vi "PS_Main.vi"() -> ()   [LabVIEW 2011]
uses:
  PS_Global.vi
  <vilib>/express/express shared/transition.llb/Dynamic To Waveform Array.vi
  <vilib>/express/express shared/transition.llb/Waveform Array To Dynamic.vi
  <vilib>/express/express arith-compare/Formula/Block/exnFormulaBlock how many pts in the wave.vi
  <vilib>/express/express shared/ex_Modify Signal Name.vi
  <vilib>/express/express arith-compare/Formula/XNode/ExpressFormulaBlockNode.xnode
panel:
  out "Std":dbl format="%#.2g%"
  out "New Value":dbl
  out "Counter":i32=1000
  out "Numbers to Avg":dbl[](array[numeric])
  in  "# in avg":i32=1000
  in  "Init Running Avg":bool
  out "Running Average":dbl format="%#.1f%"
  in  "New Discharge ON":bool
  in  "Pressure Calib":dbl=0.553
  out "LCR V Min":dbl
  in  "Discharge Voltage":dbl=10.3
  in  "Cell Pressure":dbl
  out "LCR Min V":dbl
  out "LCR Max V":dbl
  in  "stop":bool
  out "Heartbeat":string
  in  "Set All Offsets":bool
  in  "Run Polarimeter?":bool=TRUE
  out "Laser Peak Progress":i32(slide) scale=0.0..100.0
  out "Laser Global":bool
  in  "C8 Line?":bool caption="Laser State"
  out "LCR Calibration Plot":cluster{"Y":dbl[], "Y":dbl[]}[](graph)
  in  "Lower Voltge Limit":dbl=1.2
  in  "Upper Voltage Limit":dbl=4.0
  in  "Polarimeter Angle":dbl=20.0
  in  "CP In?":bool
  in  "Comment Box":string
  in  "Insert Comment":bool
  in  "Plasma On Length":dbl=0.2
  in  "Calibrate LCR":bool
  out "Plasma On":dbl
  out "Plasma State":bool caption="Plasma Ball Status"
  out "Plasma On":timestamp
  out "Shutter Closed":dbl format="%.0f sec"
  out "Shutter Time":timestamp
  in  "Shutter Set":bool=TRUE
  out "Shutter State":bool=TRUE caption="Shutter Status"
  out "log":refnum<file>
  out "VI Running":bool
  out "Off Time":timestamp
  out "On Time":timestamp
  out "Discharge State":bool caption="Discharge Status"
  out "Decay Running":bool caption="Status"
  out "Start Time":timestamp
  out "Duration":dbl
  in  "Discharge Interval":dbl=30.0
  in  "Discharge Length":dbl=5.0
  in  "Run Decay":bool
  in  "Discharge Set":bool
  out "Nuclear Polarization":dbl format="%#.1f%"
  out "Messages":string
  out "Corrected Low":dbl
  out "Corrected High":dbl
  out "Signal Offset: Laser Off":dbl
  in  "Laser State Set":bool caption="Laser State"
  out "Signal Offset: Laser On":dbl
  in  "Get Signal Offset":bool
  in  "High Signal Extend":i32
  out "Std Dev Low":dbl format="%.5f"
  out "Std Dev High":dbl format="%.5f"
  out "Optical Polarization (%)":dynamicdata(graph)
  out "Optical Polarization":dbl format="%#.1f%"
  out "Signals":dynamicdata(graph) caption="Section"
  out "Mean Low":dbl format="%.4f"
  out "Mean High":dbl format="%.4f"
  in  "High Signal Start":i32=600 caption="Begin Sample"
  in  "Low Signal Start":i32=600 caption="Begin Sample"
  out "Status":string
  out "Laser Peaks":cluster{dbl[], dbl[]}[](graph)
  out "Laser Peak Voltage Set":dbl format="%#_g V"
  in  "Run Laser Peak Find":bool
  in  "Number of Samples":i32=1000
  in  "Sample Rate (Hz)":dbl=4000.0
  # "Set Laser State"
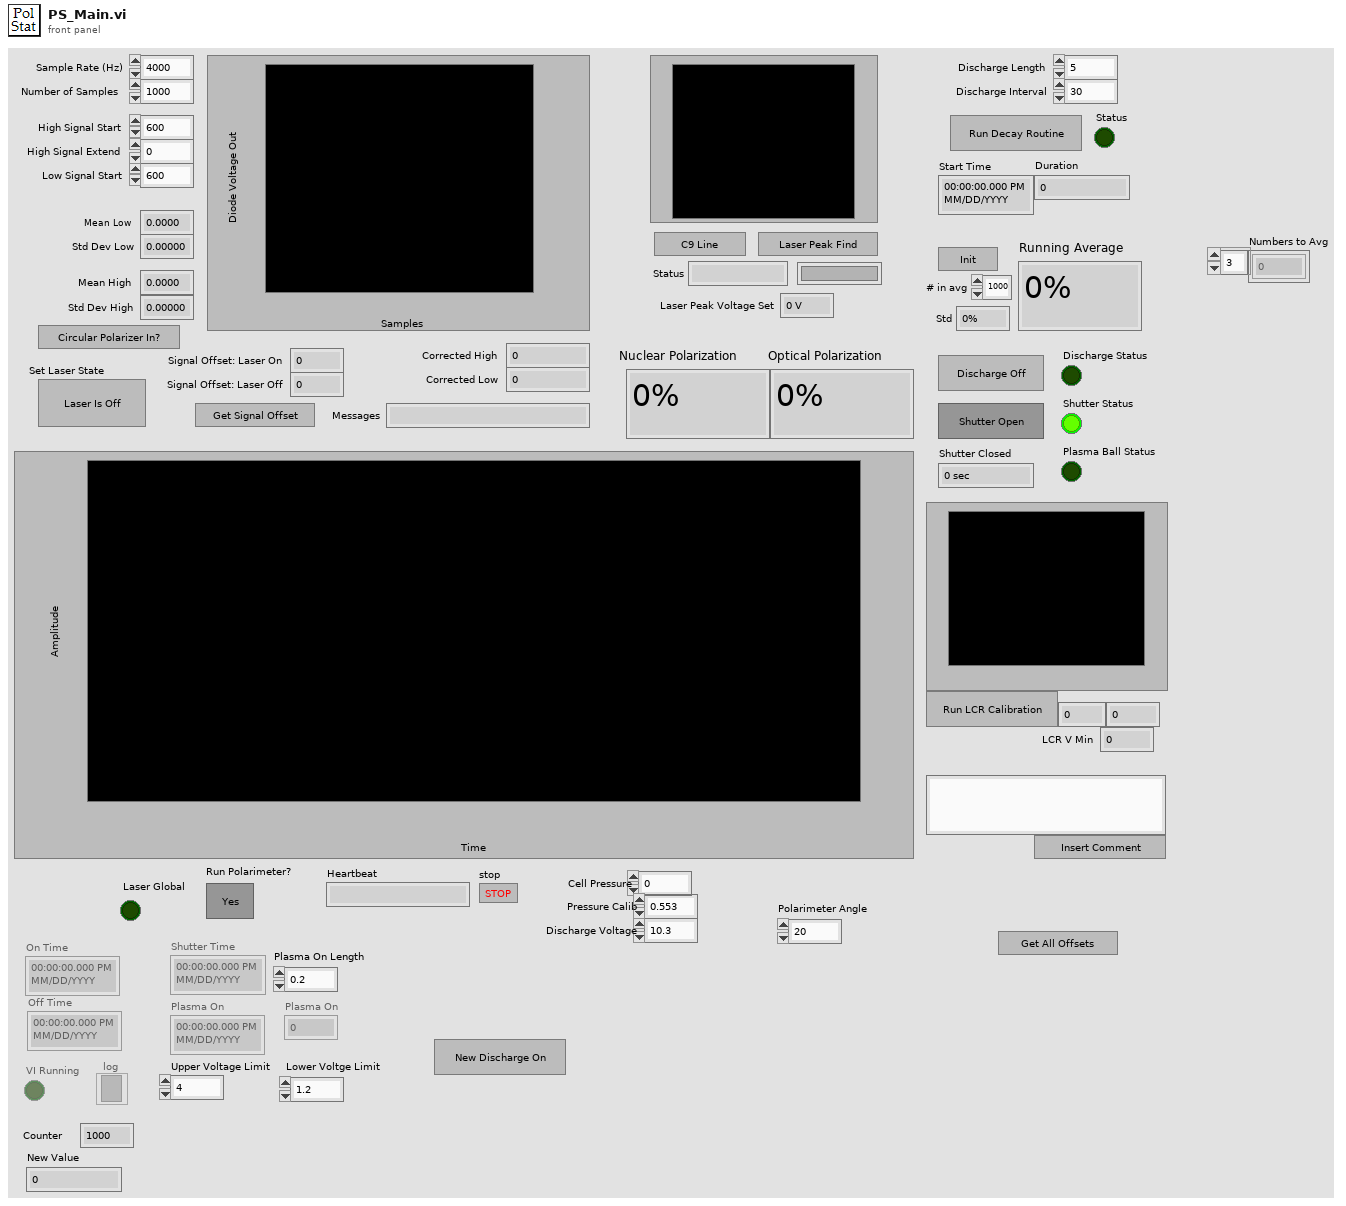
[diagram p1: front panel]
types:
  T1 = enum16{"open", "replace", "create", "open or create", "replace or create", "replace or create with confirmation"}
  T2 = enum8{"Enabled", "Disabled", "Disabled and Grayed Out"}
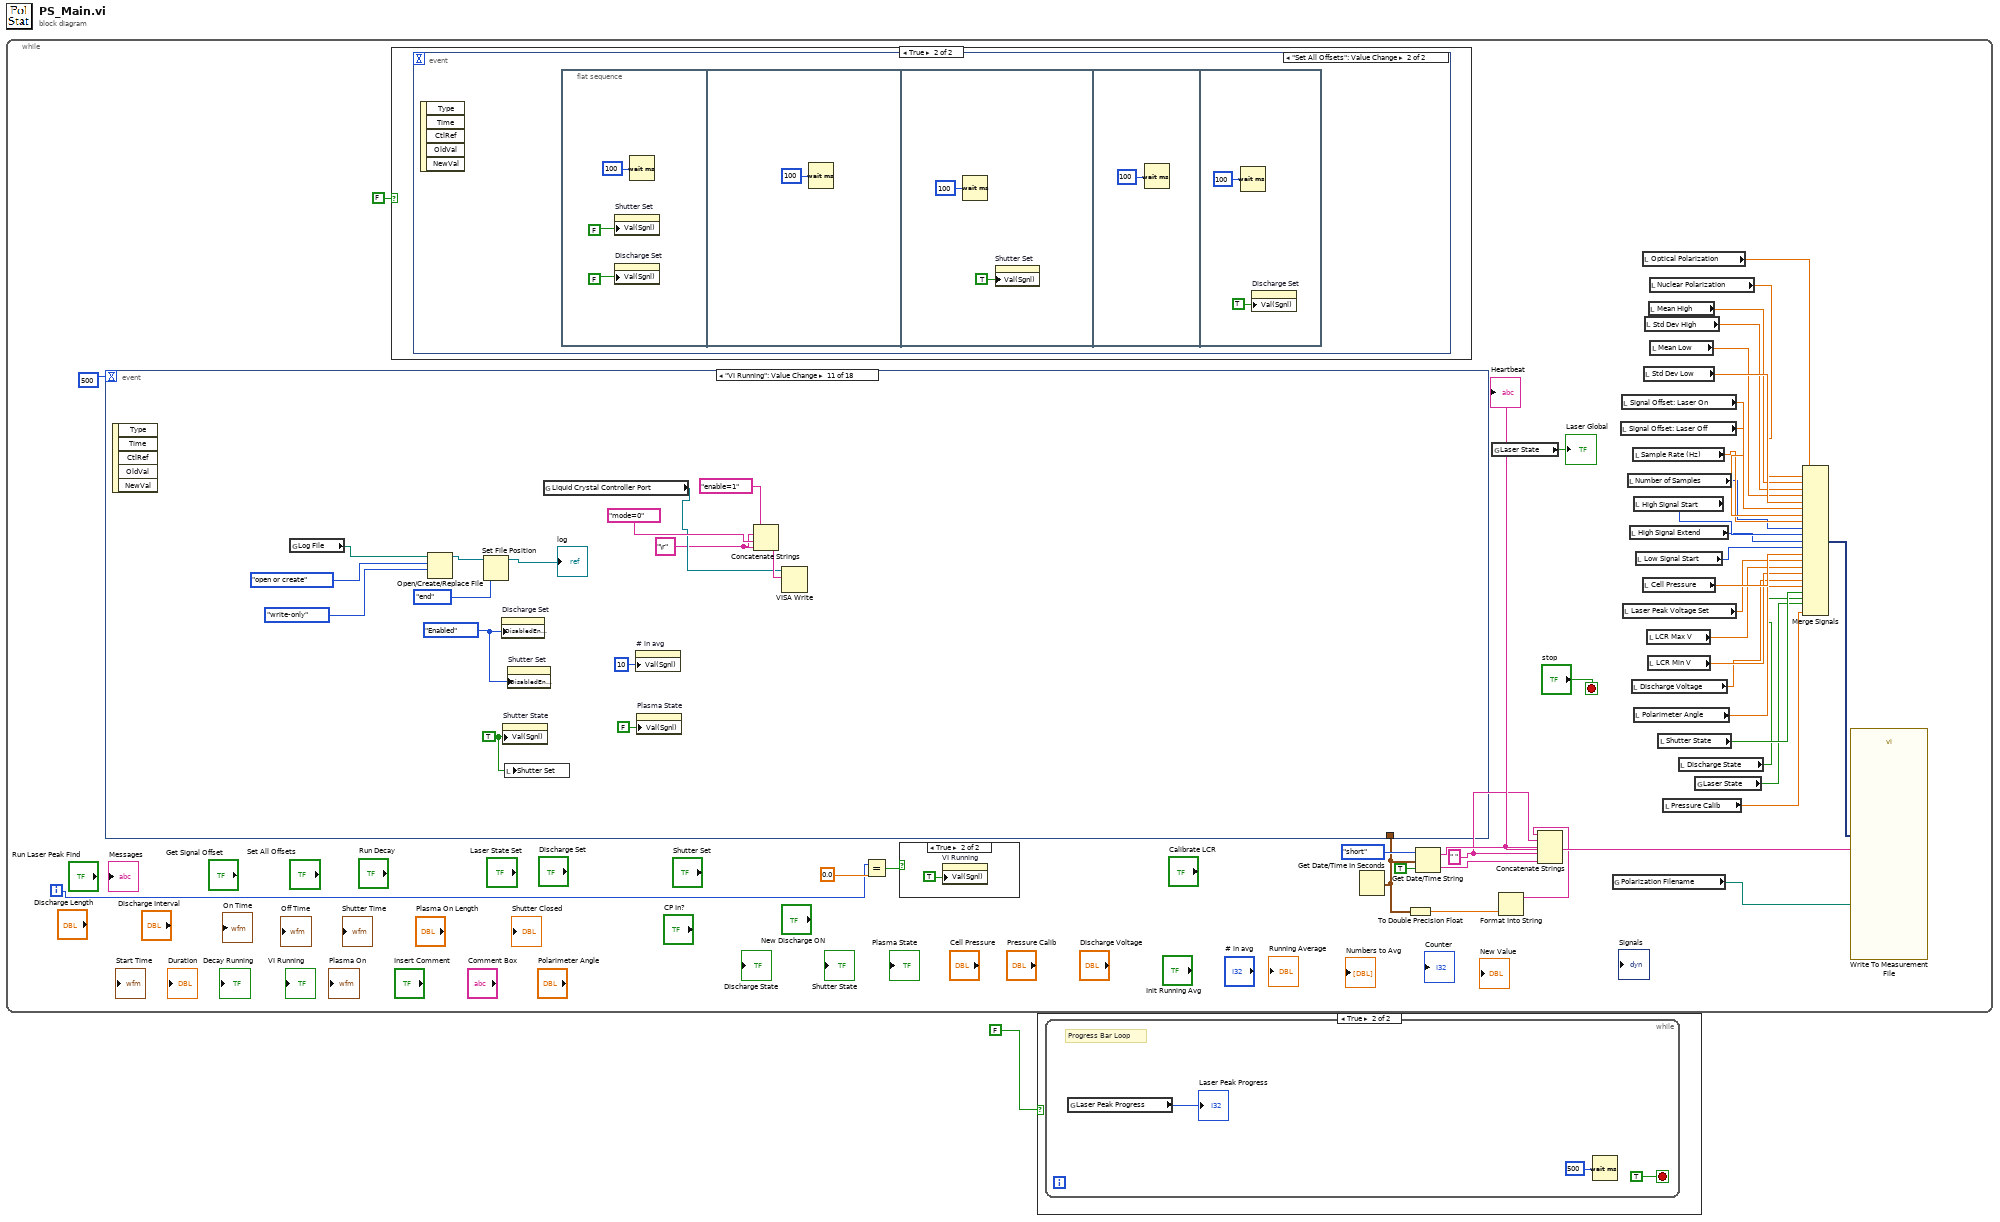
[diagram p0: block diagram]
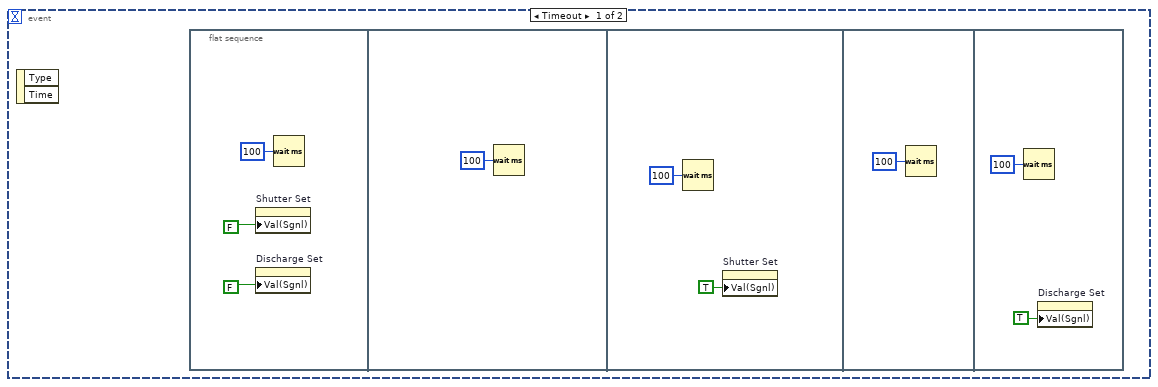
[diagram p4: hidden frame]
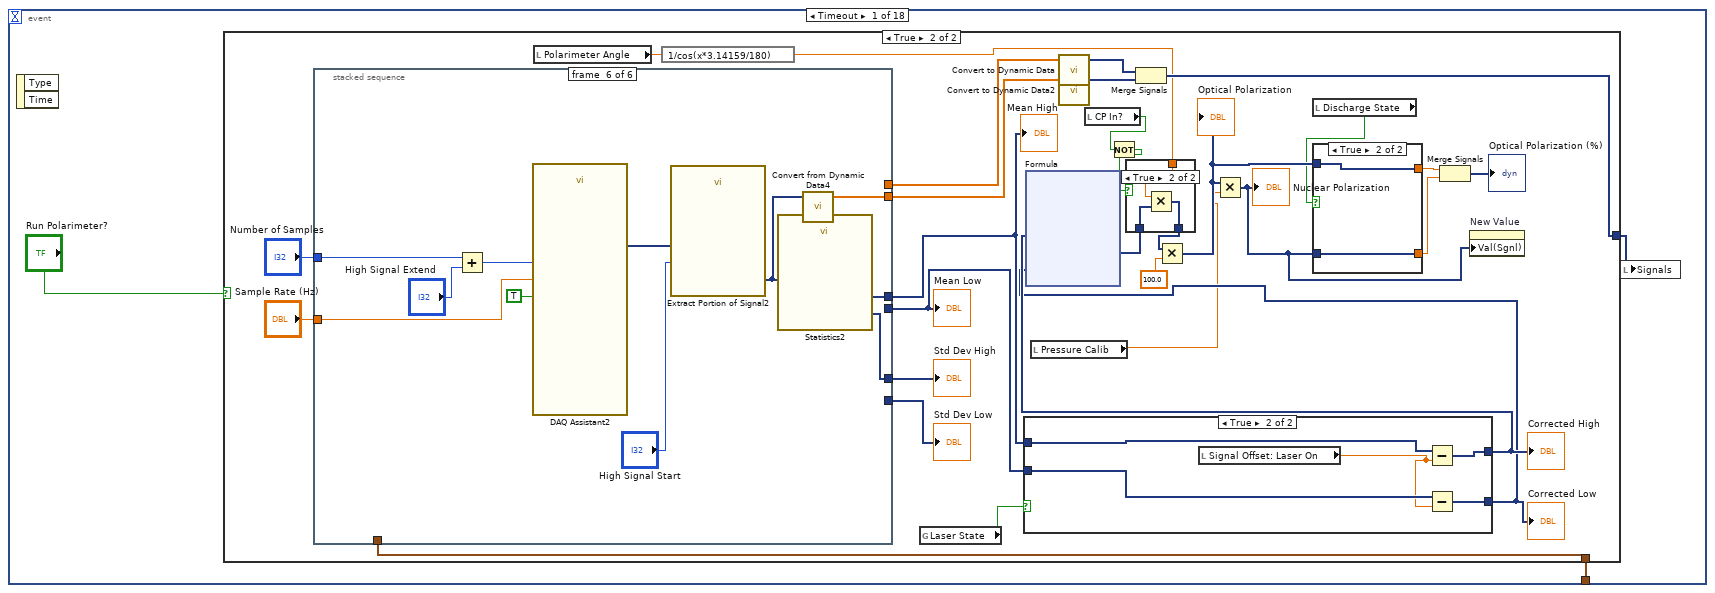
[diagram p6: hidden frame]
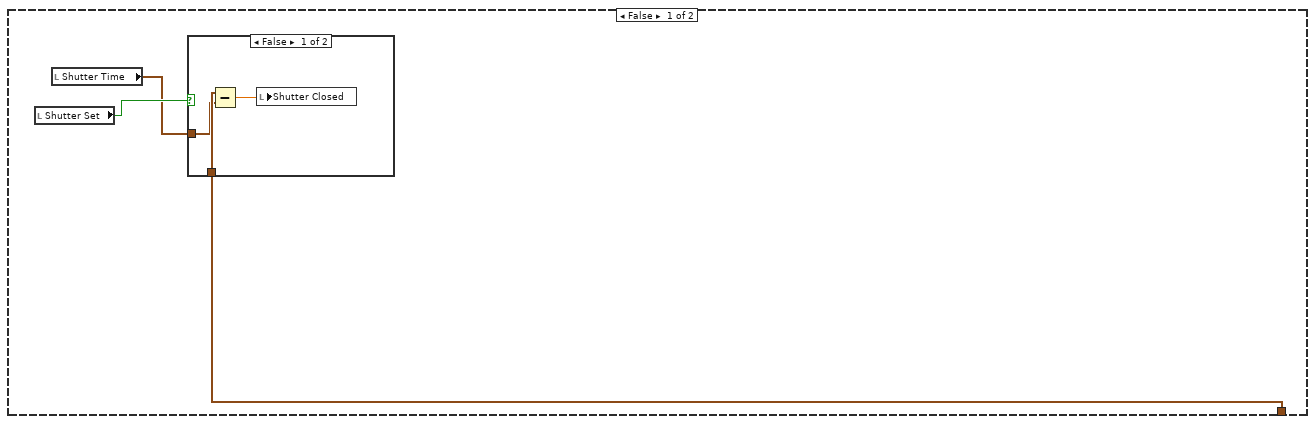
[diagram p7: hidden frame]
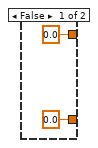
[diagram p9: hidden frame]
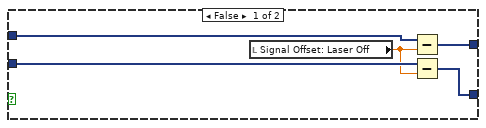
[diagram p11: hidden frame]
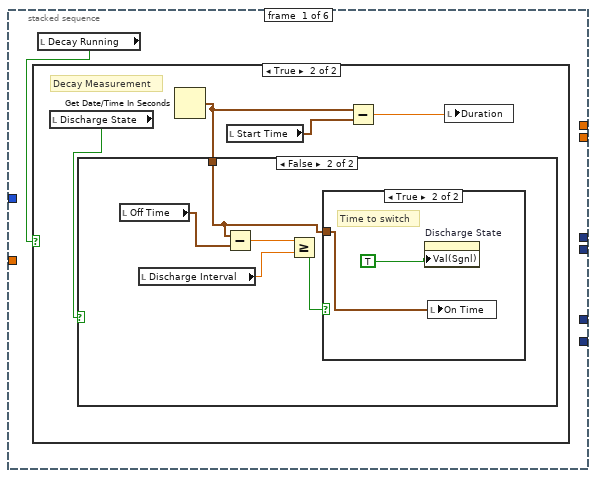
[diagram p12: hidden frame]
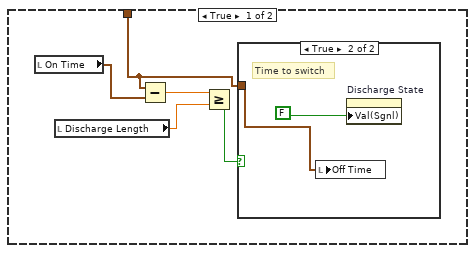
[diagram p14: hidden frame]
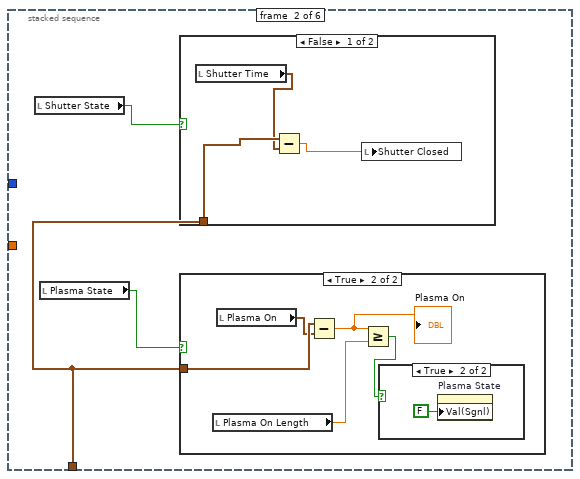
[diagram p17: hidden frame]
diagram:
  n1 = while {
    i -> [w34]
    stop <- "stop" stop-if-true
    w6 = " " ("string")
    n2 = case shown="True" FALSE {
      frame False {
      }
      frame True {
        n3 = event shown="[1] \"Set All Offsets\": Value Change" {
          selector: _ -> [_ _]
          dyn-events: _ -> [_ _]
          timeout: _ -> [_ _]
          event Timeout {
            n4 = event-data() -> ()  [unwired: 1 in, 2 out]
            n5 = flat-sequence {
              frame #0 {
                n6 = property on="Shutter Set" class="Bool (strict)"("Val(Sgnl)"=FALSE ("Value (Signaling)")) -> ()  [unwired: 2 in, 2 out]
                n7 = property on="Discharge Set" class="Bool (strict)"("Val(Sgnl)"=FALSE ("Value (Signaling)")) -> ()  [unwired: 2 in, 2 out]
                n8 = Wait (ms)(milliseconds to wait=u32 100) -> ()  [unwired: 1 out]
              }
              frame #1 {
                n9 = Wait (ms)(milliseconds to wait=u32 100) -> ()  [unwired: 1 out]
              }
              frame #2 {
                n10 = Wait (ms)(milliseconds to wait=u32 100) -> ()  [unwired: 1 out]
                n11 = property on="Shutter Set" class="Bool (strict)"("Val(Sgnl)"=TRUE ("Value (Signaling)")) -> ()  [unwired: 2 in, 2 out]
              }
              frame #3 {
                n12 = Wait (ms)(milliseconds to wait=u32 100) -> ()  [unwired: 1 out]
              }
              frame #4 {
                n13 = Wait (ms)(milliseconds to wait=u32 100) -> ()  [unwired: 1 out]
                n14 = property on="Discharge Set" class="Bool (strict)"("Val(Sgnl)"=TRUE ("Value (Signaling)")) -> ()  [unwired: 2 in, 2 out]
              }
            }
          }
          event "Set All Offsets": Value Change {
            n15 = event-data() -> ()  [unwired: 1 in, 5 out]
            n16 = flat-sequence {
              frame #0 {
                n17 = property on="Shutter Set" class="Bool (strict)"("Val(Sgnl)"=FALSE ("Value (Signaling)")) -> ()  [unwired: 2 in, 2 out]
                n18 = property on="Discharge Set" class="Bool (strict)"("Val(Sgnl)"=FALSE ("Value (Signaling)")) -> ()  [unwired: 2 in, 2 out]
                n19 = Wait (ms)(milliseconds to wait=u32 100) -> ()  [unwired: 1 out]
              }
              frame #1 {
                n20 = Wait (ms)(milliseconds to wait=u32 100) -> ()  [unwired: 1 out]
              }
              frame #2 {
                n21 = Wait (ms)(milliseconds to wait=u32 100) -> ()  [unwired: 1 out]
                n22 = property on="Shutter Set" class="Bool (strict)"("Val(Sgnl)"=TRUE ("Value (Signaling)")) -> ()  [unwired: 2 in, 2 out]
              }
              frame #3 {
                n23 = Wait (ms)(milliseconds to wait=u32 100) -> ()  [unwired: 1 out]
              }
              frame #4 {
                n24 = Wait (ms)(milliseconds to wait=u32 100) -> ()  [unwired: 1 out]
                n25 = property on="Discharge Set" class="Bool (strict)"("Val(Sgnl)"=TRUE ("Value (Signaling)")) -> ()  [unwired: 2 in, 2 out]
              }
            }
          }
        }
      }
    }
    n26 = Equal?(x=w34, y=0.0) -> (x = y?=w36:bool)
    n27 = case shown="True" w36 {
      frame False {
      }
      frame True {
        n28 = property on="VI Running" class="Bool (strict)"("Val(Sgnl)"=TRUE ("Value (Signaling)")) -> ()  [unwired: 2 in, 2 out]
      }
    }
    n29 = Get Date/Time In Seconds() -> (seconds since 1Jan1904=w9:timestamp)
    n30 = event shown="[10] \"VI Running\": Value Change" {
      selector: _ -> [_ _ _ _ _ _ _ _ _ _ _ _ _ _ _ _ _ _]
      dyn-events: _ -> [_ _ _ _ _ _ _ _ _ _ _ _ _ _ _ _ _ _]
      timeout: 500 -> [_ _ _ _ _ _ _ _ _ _ _ _ _ _ _ _ _ _]
      tunnel: w9 -> [w64 _ _ _ _ _ _ _ _ w373 _ _ _ w415 w421 _ _ _]
      event Timeout {
        n31 = event-data() -> ()  [unwired: 1 in, 2 out]
        n32 = case shown="True" "Run Polarimeter?" {
          tunnel: [_ w93] -> w62
          tunnel: w64 -> [w67 w85]
          frame False {
            n33 = local read "Shutter Set"() -> (w66:bool)
            n34 = local read "Shutter Time"() -> (w65:timestamp)
            n35 = case shown="False" w66 {
              tunnel: w67 -> [w70 _]
              tunnel: w65 -> [w68 _]
              frame False {
                n36 = Subtract(x=w70, y=w68) -> (x-y=w69:dbl)
                n37 = local write "Shutter Closed"(w69) -> ()
              }
              frame True {
              }
            }
          }
          frame True {
            n38 = stacked-sequence {
              tunnel: [_ _ _ w292 _ _] -> w97
              tunnel: "Sample Rate (Hz)" -> [_ _ _ w297 _ w309]
              tunnel: "Number of Samples" -> [_ _ _ w296 _ w301]
              tunnel: [_ _ _ _ _ w305] -> w96
              tunnel: [_ _ _ _ _ w303] -> w90
              tunnel: [_ _ _ w290 _ _] -> w88
              tunnel: [_ _ _ _ _ w302] -> w87
              tunnel: [_ _ _ w289 _ _] -> w89
              tunnel: w85 -> [_ w277 _ _ _ _]
              frame #0 {
                n39 = local read "Decay Running"() -> (w257:bool)
                n40 = case shown="True" w257 {
                  frame False {
                  }
                  frame True {
                    # "Decay Measurement"
                    n41 = local read "Discharge State"() -> (w261:bool)
                    n42 = Get Date/Time In Seconds() -> (seconds since 1Jan1904=w258:timestamp)
                    n43 = case shown="False" w261 {
                      tunnel: w258 -> [w262 w269]
                      frame True {
                        n44 = local read "On Time"() -> (w266:timestamp)
                        n45 = local read "Discharge Length"() -> (w264:dbl)
                        n46 = Subtract(x=w262, y=w266) -> (x-y=w265:dbl)
                        n47 = Greater Or Equal?(x=w265, y=w264) -> (x >= y?=w263:bool)
                        n48 = case shown="True" w263 {
                          tunnel: w262 -> [_ w268]
                          frame False {
                          }
                          frame True {
                            # "Time to switch"
                            n49 = local write "Off Time"(w268) -> ()
                            n50 = property on="Discharge State" class="Bool (strict)"("Val(Sgnl)"=FALSE) -> ()  [unwired: 2 in, 2 out]
                          }
                        }
                      }
                      frame False {
                        n51 = local read "Off Time"() -> (w273:timestamp)
                        n52 = local read "Discharge Interval"() -> (w271:dbl)
                        n53 = Subtract(x=w269, y=w273) -> (x-y=w272:dbl)
                        n54 = Greater Or Equal?(x=w272, y=w271) -> (x >= y?=w270:bool)
                        n55 = case shown="True" w270 {
                          tunnel: w269 -> [_ w275]
                          frame False {
                          }
                          frame True {
                            # "Time to switch"
                            n56 = property on="Discharge State" class="Bool (strict)"("Val(Sgnl)"=TRUE) -> ()  [unwired: 2 in, 2 out]
                            n57 = local write "On Time"(w275) -> ()
                          }
                        }
                      }
                    }
                    n58 = local read "Start Time"() -> (w259:timestamp)
                    n59 = Subtract(x=w258, y=w259) -> (x-y=w260:dbl)
                    n60 = local write "Duration"(w260) -> ()
                  }
                }
              }
              frame #1 {
                n61 = local read "Shutter State"() -> (w276:bool)
                n62 = local read "Plasma State"() -> (w278:bool)
                n63 = case shown="False" w276 {
                  tunnel: w277 -> [w287 _]
                  frame False {
                    n64 = local read "Shutter Time"() -> (w286:timestamp)
                    n65 = Subtract(x=w287, y=w286) -> (x-y=w285:dbl)
                    n66 = local write "Shutter Closed"(w285) -> ()
                  }
                  frame True {
                  }
                }
                n67 = case shown="True" w278 {
                  tunnel: w277 -> [_ w283]
                  frame False {
                  }
                  frame True {
                    n68 = local read "Plasma On Length"() -> (w279:dbl)
                    n69 = local read "Plasma On"() -> (w282:timestamp)
                    n70 = Subtract(x=w283, y=w282) -> (x-y=w281:dbl)
                    "Plasma On" <- w281
                    n71 = Greater Or Equal?(x=w281, y=w279) -> (x >= y?=w280:bool)
                    n72 = case shown="True" w280 {
                      frame False {
                      }
                      frame True {
                        n73 = property on="Plasma State" class="Bool (strict)"("Val(Sgnl)"=FALSE ("Value (Signaling)")) -> ()  [unwired: 2 in, 2 out]
                      }
                    }
                  }
                }
              }
              frame #2 {
                n74 = call "PS_LCR_Write.vi"("On/Off"=TRUE) -> ()  [unwired: 10 in, 1 out]
              }
              frame #3 {
                n75 = call "DAQ Assistant"("rate"=w297, "number of samples"=w296, "stop (F)"=TRUE) -> ("data"=w295:dynamicdata)  [unwired: 13 in, 3 out]
                n76 = call "Extract Portion of Signal"("Begin Sample"="Low Signal Start", "Signals"=w295) -> ("Section"=w291:dynamicdata)  [unwired: 8 in, 1 out]
                n77 = call "Statistics"("Signals"=w291) -> ("Standard Dev"=w289:dynamicdata, "Arithmetic Mean"=w290:dynamicdata)  [unwired: 24 in, 1 out]
                n78 = call "Convert from Dynamic Data3"("Dynamic Data Type"=w291) -> ("Array"=w292:dbl[])  [unwired: 3 in]
              }
              frame #4 {
                n79 = call "PS_LCR_Write.vi"("On/Off"=FALSE) -> ()  [unwired: 10 in, 1 out]
              }
              frame #5 {
                n80 = Add(x=w301, y="High Signal Extend") -> (x+y=w299:i32)
                n81 = call "DAQ Assistant2"("rate"=w309, "number of samples"=w299, "stop (F)"=TRUE) -> ("data"=w308:dynamicdata)  [unwired: 13 in, 3 out]
                n82 = call "Extract Portion of Signal2"("Begin Sample"="High Signal Start", "Signals"=w308) -> ("Section"=w304:dynamicdata)  [unwired: 8 in, 1 out]
                n83 = call "Statistics2"("Signals"=w304) -> ("Standard Dev"=w302:dynamicdata, "Arithmetic Mean"=w303:dynamicdata)  [unwired: 24 in, 1 out]
                n84 = call "Convert from Dynamic Data4"("Dynamic Data Type"=w304) -> ("Array"=w305:dbl[])  [unwired: 3 in]
              }
            }
            "Mean High" <- w90
            "Mean Low" <- w88
            "Std Dev High" <- w87
            "Std Dev Low" <- w89
            n85 = local read "Polarimeter Angle"() -> (w82:dbl)
            n86 = expression code="1/cos(x*3.14159/180)"(w82) -> (w81:dbl)
            n87 = global read "PS_Global.vi" "Laser State"() -> (w86:bool)
            n88 = case shown="True" w86 {
              tunnel: w88 -> [w249 w253]
              tunnel: w90 -> [w251 w254]
              tunnel: [w250 w256] -> w78
              tunnel: [w248 w255] -> w77
              frame False {
                n89 = local read "Signal Offset: Laser Off"() -> (w247:dbl)
                n90 = Subtract(x=w251, y=w247) -> (x-y=w250:dynamicdata)
                n91 = Subtract(x=w249, y=w247) -> (x-y=w248:dynamicdata)
              }
              frame True {
                n92 = local read "Signal Offset: Laser On"() -> (w252:dbl)
                n93 = Subtract(x=w254, y=w252) -> (x-y=w256:dynamicdata)
                n94 = Subtract(x=w253, y=w252) -> (x-y=w255:dynamicdata)
              }
            }
            "Corrected High" <- w78
            "Corrected Low" <- w77
            n95 = xnode "Formula"("X1"=w78, "X2"=w77) -> ("Result"=w84:dynamicdata)  [unwired: 1 in, 1 out]
            n96 = local read "Pressure Calib"() -> (w73:dbl)
            n97 = call "Convert to Dynamic Data"("Array"=w97) -> ("Dynamic Data Type"=w95:dynamicdata)  [unwired: 3 in]
            n98 = call "Convert to Dynamic Data2"("Array"=w96) -> ("Dynamic Data Type"=w94:dynamicdata)  [unwired: 3 in]
            n99 = local read "CP In?"() -> (w80:bool)
            n100 = Not(x=w80) -> (.not. x?=w79:bool)
            n101 = case shown="True" w79 {
              tunnel: w84 -> [w104 w107]
              tunnel: [w104 w106] -> w83
              tunnel: w81 -> [_ w105]
              frame False {
              }
              frame True {
                n102 = Multiply(x=w105, y=w107) -> (x*y=w106:dynamicdata)
              }
            }
            n103 = Merge Signals(w95, w94) -> (w93:dynamicdata)
            n104 = Multiply(x=w83, y=100.0) -> (x*y=w76:dynamicdata)
            "Optical Polarization" <- w76
            n105 = Multiply(x=w76, y=w73) -> (x*y=w71:dynamicdata)
            "Nuclear Polarization" <- w71
            n106 = local read "Discharge State"() -> (w74:bool)
            n107 = case shown="True" w74 {
              tunnel: [0.0 w103] -> w72
              tunnel: w76 -> [_ w103]
              tunnel: w71 -> [_ w102]
              tunnel: [0.0 w102] -> w75
              frame False {
              }
              frame True {
              }
            }
            n108 = Merge Signals(w72, w75) -> (→"Optical Polarization (%)":dynamicdata)
            n109 = property on="New Value" class="DigNum (strict)"("Val(Sgnl)"=w71) -> ()  [unwired: 2 in, 2 out]
          }
        }
        n110 = local write "Signals"(w62) -> ()
      }
      event "Init Running Avg", "Numbers to Avg": Value Change {
        n111 = event-data() -> ()  [unwired: 1 in, 5 out]
        n112 = local read "# in avg"() -> (w313:i32)
        n113 = Initialize Array(0.0 ("element"), w313) -> (w311:dbl[])
        n114 = local write "Counter"(0 ("Counter")) -> ()
        n115 = local write "Numbers to Avg"(w311) -> ()
      }
      event "New Value": Value Change {
        n116 = event-data() -> ("NewVal"=w315:dbl)  [unwired: 1 in, 4 out]
        n117 = flat-sequence {
          tunnel: w315 -> [w323]
          tunnel: [w321] -> w314
          tunnel: w314 -> [w325]
          frame #0 {
            n118 = local read "Numbers to Avg"() -> (w322:dbl[])
            n119 = local read "Counter"() -> (w321:i32)
            n120 = local read "# in avg"() -> (w324:i32)
            n121 = Quotient & Remainder(x=w321, y=w324) -> (x-y*floor(x/y)=w320:i32)  [unwired: 1 out]
            n122 = Replace Array Subset(array=w322, new element=w323, index=w320) -> (w319:dbl[])
            n123 = call "Convert to Dynamic Data3"("Array"=w319) -> ("Dynamic Data Type"=w318:dynamicdata)  [unwired: 3 in]
            n124 = call "Statistics4"("Signals"=w318) -> ("Standard Dev"=→"Std":dynamicdata, "Arithmetic Mean"=w317:dynamicdata)  [unwired: 24 in, 1 out]
            n125 = local write "Numbers to Avg"(w319) -> ()
            n126 = local write "Running Average"(w317) -> ()
          }
          frame #1 {
            n127 = Increment(x=w325) -> (x+1=w326:i32)
            n128 = local write "Counter"(w326) -> ()
          }
        }
      }
      event "New Discharge ON": Value Change {
        n129 = event-data() -> ()  [unwired: 1 in, 5 out]
      }
      event "Cell Pressure": Value Change {
        n130 = event-data() -> ("NewVal"=w332:dbl)  [unwired: 1 in, 4 out]
        n131 = call "PS_Pressure_Cal.vi"("P"=w332) -> ("Pn"=w329:dbl)  [unwired: 9 in, 1 out]
        n132 = local write "Pressure Calib"(w329) -> ()
        n133 = Format Into String(format string="%.2f", w332) -> (resulting string=w335:string)  [unwired: 2 in, 1 out]
        n134 = Format Into String(format string="%.2f", w329) -> (resulting string=w330:string)  [unwired: 2 in, 1 out]
        n135 = Concatenate Strings("Pressure: " ("Messages"), w335, " torr gives " ("string"), w330, "." ("string")) -> (w327:string)
        n136 = property on="Messages" class="Str"("Val(Sgnl)"=w327) -> ()  [unwired: 2 in, 2 out]
      }
      event "Insert Comment": Value Change {
        n137 = event-data() -> ()  [unwired: 1 in, 5 out]
        n138 = local read "Comment Box"() -> (w338:string)
        n139 = local write "Insert Comment"(FALSE ("Insert Comment")) -> ()
        n140 = property on="Messages" class="Str"("Val(Sgnl)"=w338) -> ()  [unwired: 2 in, 2 out]
      }
      event "Calibrate LCR": Value Change {
        n141 = event-data() -> ("NewVal"=w339:bool)  [unwired: 1 in, 4 out]
        n142 = case shown="True" w339 {
          frame False {
          }
          frame True {
            n143 = flat-sequence {
              frame #0 {
                n144 = global write "PS_Global.vi" "Calibration Progress"(u8 0 ("Calibration Progress")) -> ()
                n145 = call "PS_LCR_cal.vi"("Lower Voltge Limit"="Lower Voltge Limit", "Upper Voltage Limit"="Upper Voltage Limit") -> ("Min"=→"LCR V Min":dbl, "XY Graph"=→"LCR Calibration Plot":cluster{"Y":dbl[], "Y":dbl[]}[], "Min Voltage"=→"LCR Min V":dbl, "Max Voltage"=→"LCR Max V":dbl)  [unwired: 6 in]
                n146 = property on="Discharge Set" class="Bool (strict)"("Val(Sgnl)"=TRUE ("Value (Signaling)")) -> ()  [unwired: 2 in, 2 out]
              }
              frame #1 {
                n147 = global write "PS_Global.vi" "Laser Peak Progress"(u8 100 ("Laser Peak Progress")) -> ()
                n148 = property on="Calibrate LCR" class="Bool (strict)"("Val(Sgnl)"=FALSE ("Value (Signaling)")) -> ()  [unwired: 2 in, 2 out]
              }
            }
          }
        }
        n149 = property on="Calibrate LCR" class="Bool (strict)"("Blinking"=w339) -> ()  [unwired: 2 in, 2 out]
      }
      event "Laser State Set": Value Change {
        n150 = event-data() -> ("NewVal"=w351:bool)  [unwired: 1 in, 4 out]
        n151 = local read "Shutter State"() -> (w350:bool)
        n152 = And(x=w350, y=w351) -> (x .and. y?=w352:bool)
        n153 = global write "PS_Global.vi" "Laser State"(w352) -> ()
      }
      event "Get Signal Offset": Value Change {
        n154 = event-data() -> ()  [unwired: 1 in, 5 out]
        n155 = call "DAQ Assistant3"("rate"=1000.0, "number of samples"=2000, "stop (F)"=TRUE) -> ("data"=w355:dynamicdata)  [unwired: 13 in, 3 out]
        n156 = global read "PS_Global.vi" "Laser State"() -> (w354:bool)
        n157 = call "Statistics3"("Signals"=w355) -> ("Arithmetic Mean"=w353:dynamicdata)  [unwired: 24 in, 2 out]
        n158 = case shown="False" w354 {
          tunnel: w353 -> [w365 w367]
          tunnel: ["Laser off " ("string") "Laser on " ("string")] -> w359
          frame False {
            "Signal Offset: Laser Off" <- w365
          }
          frame True {
            "Signal Offset: Laser On" <- w367
          }
        }
        n159 = Format Into String(format string="%.4f", w353) -> (resulting string=w358:string)  [unwired: 2 in, 1 out]
        n160 = Concatenate Strings(w359, "signal offset set to " ("string"), w358) -> (w356:string)
        n161 = property on="Messages" class="Str"("Val(Sgnl)"=w356) -> ()  [unwired: 2 in, 2 out]
        n162 = local write "Signals"(w353) -> ()
      }
      event "Messages": Value Change {
        n163 = event-data() -> ("NewVal"=w372:string)  [unwired: 1 in, 4 out]
        n164 = call <vilib>:"Space Constant.vi"() -> ("String"=w368:string)
        n165 = Get Date/Time String(date format (0)=enum16{"short", "long", "abbreviated"}."short", seconds (now)=w373, want seconds? (F)=TRUE) -> (date string=w376:string, time string=w377:string)
        n166 = local read "log"() -> (w371:refnum<file>)
        n167 = Concatenate Strings(w376, w368, w377, w368, w372, "\r") -> (w370:string)
        n168 = Write to Text File(file (use dialog)=w371, text=w370) -> ()  [unwired: 2 in, 3 out]
      }
      event "VI Running": Value Change {
        w380 = "\r"
        w388 = TRUE ("Value (Signaling)")
        w389 = T2."Enabled" ("Disabled")
        n169 = event-data() -> ()  [unwired: 1 in, 5 out]
        n170 = global read "PS_Global.vi" "Log File"() -> (w392:path)
        n171 = Open/Create/Replace File(file path (use dialog)=w392, operation (0:open)=T1."open or create", access (0:read/write)=enum16{"read/write", "read-only", "write-only"}."write-only") -> (refnum out=w386:refnum<file>)  [unwired: 3 in, 2 out]
        n172 = Set File Position(refnum=w386, from (0:start)=enum16{"start", "end", "current"}."end") -> (refnum out=→"log":refnum<file>)  [unwired: 2 in, 1 out]
        n173 = property on="Discharge Set" class="Bool (strict)"("DisabledEnum"=w389) -> ()  [unwired: 2 in, 2 out]
        n174 = property on="Shutter State" class="Bool (strict)"("Val(Sgnl)"=w388) -> ()  [unwired: 2 in, 2 out]
        n175 = local write "Shutter Set"(w388) -> ()
        n176 = property on="Shutter Set" class="Bool (strict)"("DisabledEnum"=w389) -> ()  [unwired: 2 in, 2 out]
        n177 = global read "PS_Global.vi" "Liquid Crystal Controller Port"() -> (w381:refnum<visa-resource-name>)
        n178 = property on="# in avg" class="DigNum (strict)"("Val(Sgnl)"=10 ("Value (Signaling)")) -> ()  [unwired: 2 in, 2 out]
        n179 = property on="Plasma State" class="Bool (strict)"("Val(Sgnl)"=FALSE ("Value (Signaling)")) -> ()  [unwired: 2 in, 2 out]
        n180 = Concatenate Strings("enable=1" ("write buffer"), w380, "mode=0" ("write buffer"), w380) -> (w383:string)
        n181 = VISA Write(VISA resource name=w381, write buffer=w383) -> ()  [unwired: 1 in, 3 out]
      }
      event "Run Laser Peak Find": Value Change {
        n182 = event-data() -> ()  [unwired: 1 in, 5 out]
        n183 = flat-sequence {
          tunnel: [w399] -> w394
          tunnel: ["C8 Line?"] -> w393
          tunnel: w394 -> [w407]
          tunnel: w393 -> [w402]
          frame #0 {
            n184 = global write "PS_Global.vi" "Laser Peak Progress"(u8 0 ("Laser Peak Progress")) -> ()
            n185 = local write "Status"("Running" ("Status")) -> ()
            n186 = property on="Status" class="Str"("Blinking"=TRUE) -> ()  [unwired: 2 in, 2 out]
          }
          frame #1 {
            n187 = call "PS_Laser_Set.vi"("C8 Line?"="C8 Line?") -> ("XY Graph"=→"Laser Peaks":cluster{dbl[], dbl[]}[], "Voltage Set To"=w399:dbl)  [unwired: 8 in]
            "Laser Peak Voltage Set" <- w399
          }
          frame #2 {
            n188 = property on="Status" class="Str"("Blinking"=FALSE) -> ()  [unwired: 2 in, 2 out]
            n189 = local write "Status"("Done!" ("Status")) -> ()
            n190 = case shown="False" w402 {
              tunnel: ["C9 line." ("Messages") "C8 line." ("Messages")] -> w401
              frame False {
              }
              frame True {
              }
            }
            n191 = Format Into String(format string="%.2f", w407) -> (resulting string=w406:string)  [unwired: 2 in, 1 out]
            n192 = Concatenate Strings("Set Laser Peak to " ("Messages"), w406, " V, " ("string"), w401) -> (w403:string)
            n193 = property on="Messages" class="Str"("Val(Sgnl)"=w403) -> ()  [unwired: 2 in, 2 out]
          }
        }
      }
      event "Discharge State": Value Change {
        n194 = event-data() -> ("NewVal"=w413:bool)  [unwired: 1 in, 4 out]
        n195 = call "PS_Discharge_Control.vi"("On/Off"=w413) -> ()  [unwired: 10 in, 1 out]
        n196 = property on="Plasma State" class="Bool (strict)"("Val(Sgnl)"=w413) -> ()  [unwired: 2 in, 2 out]
      }
      event "Plasma State": Value Change {
        n197 = event-data() -> ("NewVal"=w414:bool)  [unwired: 1 in, 4 out]
        n198 = case shown="True" w414 {
          tunnel: w415 -> [_ w416]
          frame False {
          }
          frame True {
            n199 = local write "Plasma On"(w416) -> ()
          }
        }
        n200 = call "PS_Plasma_Ball.vi"("On/Off"=w414) -> ()  [unwired: 10 in, 1 out]
      }
      event "Shutter State": Value Change {
        n201 = event-data() -> ("NewVal"=w419:bool)  [unwired: 1 in, 4 out]
        n202 = local read "Laser State Set"() -> (w418:bool)
        n203 = Not(x=w419) -> (.not. x?=w420:bool)
        n204 = call "PS_Shutter_Control.vi"("On/Off"=w419) -> ()  [unwired: 10 in, 1 out]
        n205 = property on="Shutter Closed" class="DigNum (strict)"("Blinking"=w420) -> ()  [unwired: 2 in, 2 out]
        n206 = And(x=w419, y=w418) -> (x .and. y?=w417:bool)
        n207 = global write "PS_Global.vi" "Laser State"(w417) -> ()
        n208 = case shown="True" w420 {
          tunnel: w421 -> [_ w422]
          frame False {
          }
          frame True {
            n209 = local write "Shutter Time"(w422) -> ()
          }
        }
      }
      event "Run Decay": Value Change {
        n210 = event-data() -> ("NewVal"=w424:bool)  [unwired: 1 in, 4 out]
        n211 = case shown="True" w424 {
          frame False {
            w429 = T2."Enabled" ("Disabled")
            # "Stopping: set discharge and shutter to button state"
            n212 = property on="Discharge Set" class="Bool (strict)"("DisabledEnum"=w429) -> ()  [unwired: 2 in, 2 out]
            n213 = property on="Shutter Set" class="Bool (strict)"("DisabledEnum"=w429) -> ()  [unwired: 2 in, 2 out]
            n214 = local write "Decay Running"(FALSE ("Decay Running")) -> ()
            n215 = local read "Discharge Set"() -> (w431:bool)
            n216 = local read "Shutter Set"() -> (w430:bool)
            n217 = property on="Shutter State" class="Bool (strict)"("Val(Sgnl)"=w430) -> ()  [unwired: 2 in, 2 out]
            n218 = property on="Discharge State" class="Bool (strict)"("Val(Sgnl)"=w431) -> ()  [unwired: 2 in, 2 out]
          }
          frame True {
            w434 = FALSE ("Discharge State")
            w435 = T2."Disabled and Grayed Out" ("Disabled")
            # "Starting: Turn off discharge, close laser shutter"
            n219 = Get Date/Time In Seconds() -> (seconds since 1Jan1904=w433:timestamp)
            n220 = local write "Duration"(0.0 ("Duration")) -> ()
            n221 = local write "Decay Running"(TRUE ("Laser State 2")) -> ()
            n222 = property on="Discharge Set" class="Bool (strict)"("DisabledEnum"=w435) -> ()  [unwired: 2 in, 2 out]
            n223 = property on="Shutter Set" class="Bool (strict)"("DisabledEnum"=w435) -> ()  [unwired: 2 in, 2 out]
            n224 = local write "Start Time"(w433) -> ()
            n225 = property on="Discharge State" class="Bool (strict)"("Val(Sgnl)"=w434) -> ()  [unwired: 2 in, 2 out]
            n226 = property on="Shutter State" class="Bool (strict)"("Val(Sgnl)"=w434) -> ()  [unwired: 2 in, 2 out]
          }
        }
        n227 = case shown="True" w424 {
          tunnel: ["stopped." ("string") "started." ("string")] -> w425
          frame False {
          }
          frame True {
          }
        }
        n228 = Concatenate Strings("Decay routine " ("string"), w425) -> (w423:string)
        n229 = property on="Messages" class="Str"("Val(Sgnl)"=w423) -> ()  [unwired: 2 in, 2 out]
      }
      event "Discharge Set": Value Change {
        n230 = event-data() -> ("NewVal"=w439:bool)  [unwired: 1 in, 4 out]
        n231 = case shown="True" w439 {
          tunnel: ["off." ("string") "on." ("string")] -> w440
          frame False {
          }
          frame True {
          }
        }
        n232 = Concatenate Strings("Discharge turned " ("string"), w440) -> (w438:string)
        n233 = property on="Discharge State" class="Bool (strict)"("Val(Sgnl)"=w439) -> ()  [unwired: 2 in, 2 out]
        n234 = property on="Messages" class="Str"("Val(Sgnl)"=w438) -> ()  [unwired: 2 in, 2 out]
      }
      event "Shutter Set": Value Change {
        n235 = event-data() -> ("NewVal"=w444:bool)  [unwired: 1 in, 4 out]
        n236 = case shown="False" w444 {
          tunnel: ["closed." ("string") "opened." ("string")] -> w446
          frame False {
          }
          frame True {
          }
        }
        n237 = Concatenate Strings("Shutter " ("string"), w446) -> (w445:string)
        n238 = property on="Messages" class="Str"("Val(Sgnl)"=w445) -> ()  [unwired: 2 in, 2 out]
        n239 = property on="Shutter State" class="Bool (strict)"("Val(Sgnl)"=w444) -> ()  [unwired: 2 in, 2 out]
      }
    }
    n240 = To Double Precision Float(number=w9) -> (double precision float=w8:dbl)
    n241 = Get Date/Time String(date format (0)=enum16{"short", "long", "abbreviated"}."short", seconds (now)=w9, want seconds? (F)=TRUE) -> (date string=w39:string, time string=w38:string)
    n242 = global read "PS_Global.vi" "Laser State"() -> (→"Laser Global":bool)
    n243 = Format Into String(w8) -> (resulting string=w7:string)  [unwired: 3 in, 1 out]
    n244 = Concatenate Strings(w7, w6, w39, w6, w38) -> (w37:string)
    "Heartbeat" <- w37
    n245 = global read "PS_Global.vi" "Polarization Filename"() -> (w2:path)
    n246 = local read "Signal Offset: Laser Off"() -> (w29:dbl)
    n247 = local read "Signal Offset: Laser On"() -> (w30:dbl)
    n248 = local read "Laser Peak Voltage Set"() -> (w22:dbl)
    n249 = local read "Number of Samples"() -> (w27:i32)
    n250 = local read "High Signal Extend"() -> (w25:i32)
    n251 = local read "Discharge Voltage"() -> (w19:dbl)
    n252 = local read "Sample Rate (Hz)"() -> (w28:dbl)
    n253 = local read "High Signal Start"() -> (w26:i32)
    n254 = local read "Polarimeter Angle"() -> (w17:dbl)
    n255 = local read "Low Signal Start"() -> (w24:i32)
    n256 = local read "Optical Polarization"() -> (w10:dbl)
    n257 = local read "Cell Pressure"() -> (w23:dbl)
    n258 = local read "Std Dev Low"() -> (w15:dbl)
    n259 = local read "Std Dev High"() -> (w13:dbl)
    n260 = local read "LCR Max V"() -> (w21:dbl)
    n261 = local read "LCR Min V"() -> (w20:dbl)
    n262 = local read "Mean High"() -> (w12:dbl)
    n263 = local read "Nuclear Polarization"() -> (w11:dbl)
    n264 = local read "Mean Low"() -> (w14:dbl)
    n265 = local read "Shutter State"() -> (w16:bool)
    n266 = local read "Pressure Calib"() -> (w3:dbl)
    n267 = local read "Discharge State"() -> (w5:bool)
    n268 = global read "PS_Global.vi" "Laser State"() -> (w4:bool)
    n269 = Merge Signals(w10, w11, w12, w13, w14, w15, w30, w29, w28, w27, w26, w25, w24, w23, w22, w21, w20, w19, w17, w16, w5, w4, w3) -> (w18:dynamicdata)
    n270 = call "Write To Measurement File"("Signals"=w18, "Filename"=w2, "Comment"=w37) -> ()  [unwired: 14 in, 3 out]
  }
  n271 = case shown="True" FALSE {
    frame False {
    }
    frame True {
      n272 = while {
        stop <- TRUE stop-if-true
        # "Progress Bar Loop"
        n273 = global read "PS_Global.vi" "Laser Peak Progress"() -> (→"Laser Peak Progress":u8)
        n274 = Wait (ms)(milliseconds to wait=u32 500) -> ()  [unwired: 1 out]
      }
    }
  }
